vi "Process Heartbeat Waveform.vi"(7 "Pressure Measurement":dbl, 8 "error in (no error)":errorcluster, 11 "Heart Rate Params":T1={"Heart Rates"=[], "Peak Pressures"=[], "Peak Amplitudes"=[], "History Length"=20, "Last  Slope"=20.0, "filtered history"=[], "raw history"=[], "Pulse"=FALSE, "Heart Rate Timer"=0, "Iteration"=0, "Pressure of Valley"=0.0, "Slope Log"=[], "Signal Segment"=refnum, "Acquisition Graph"=refnum, "This VI"=refnum, "Name"=""}) -> (0 "error out":errorcluster, 1 "BPM":dbl, 2 "Last Slope":dbl(graph), 3 "Heart Rate Params Out":T1 caption="Heart Rate Params 2", 5 "Pulse":bool)   [LabVIEW 2017]
doc: "[Covers: SoftwareReq5]"
uses:
  Custom Controls/Heart Rate Parameters.ctl
panel:
  out "history":dbl[](array[numeric])
  out "Peak pressure":dbl
  out "Pressure":dbl
  out "Pressure low":dbl
  out "Slope":dbl
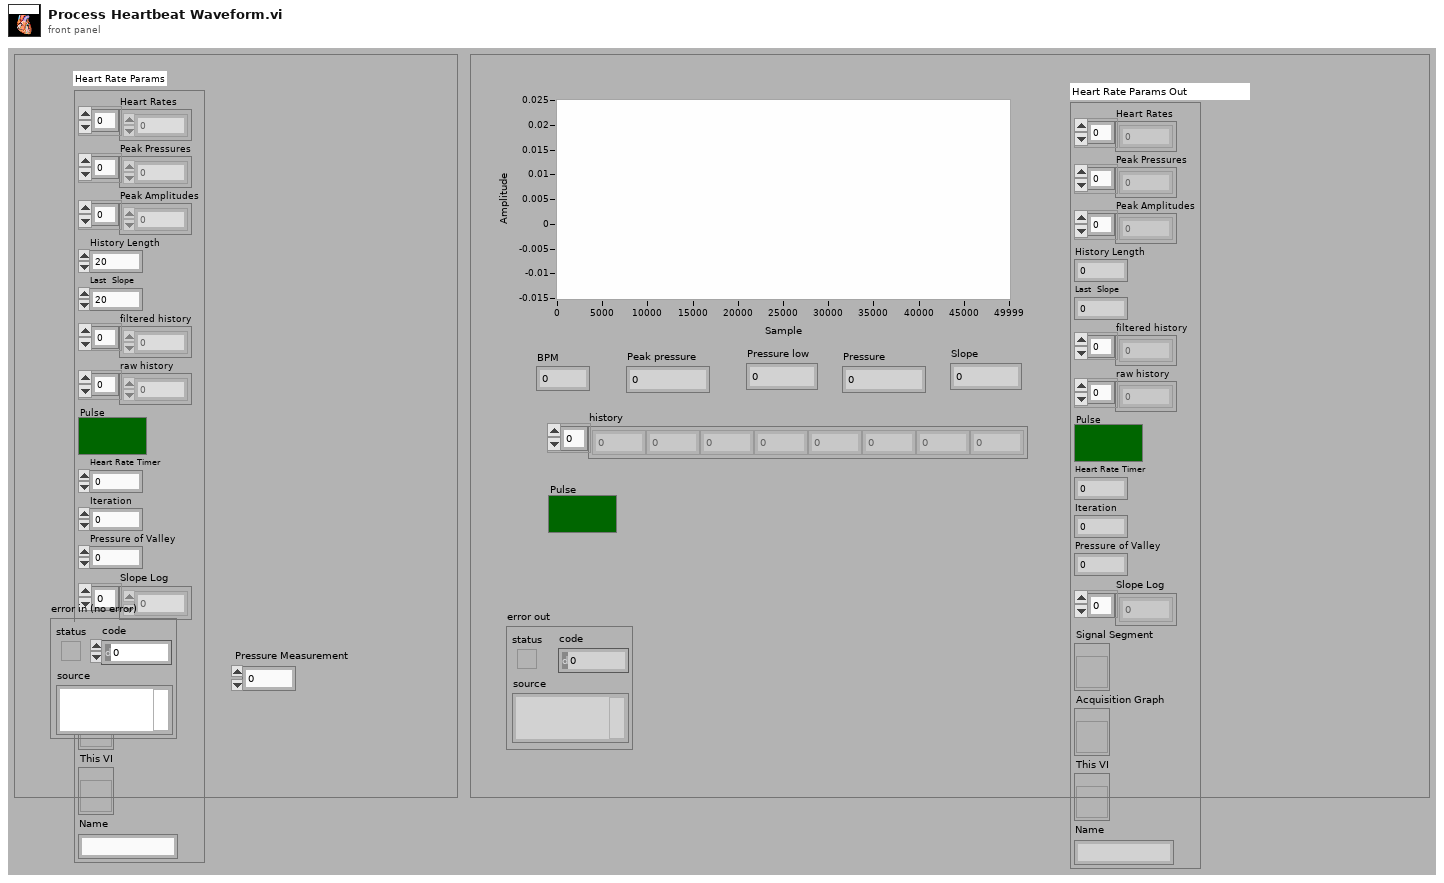
[diagram p1: front panel]
types:
  T1 = typedef "Heart Rate Parameters.ctl" = cluster{"Heart Rates":dbl[], "Peak Pressures":dbl[], "Peak Amplitudes":dbl[], "History Length":i32, "Last  Slope":dbl, "filtered history":dbl[], "raw history":dbl[], "Pulse":bool, "Heart Rate Timer":i32, "Iteration":u32, "Pressure of Valley":dbl, "Slope Log":dbl[], "Signal Segment":refnum<vi>, "Acquisition Graph":refnum<vi>, "This VI":refnum<vi>, "Name":string}
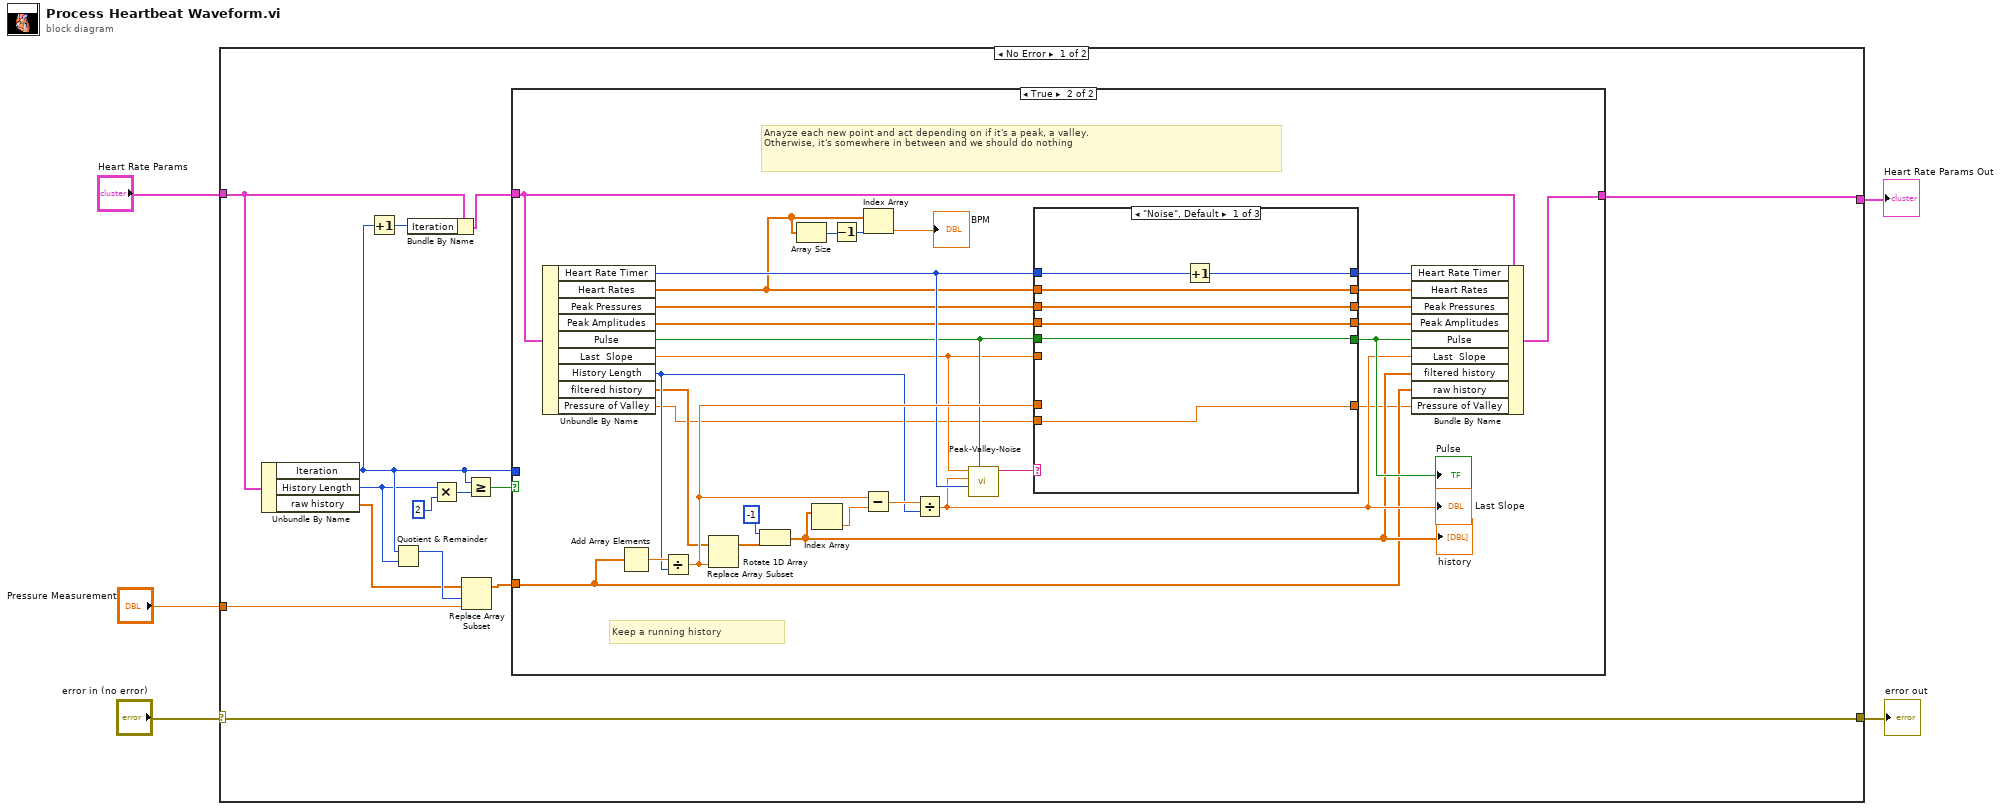
[diagram p0: block diagram]
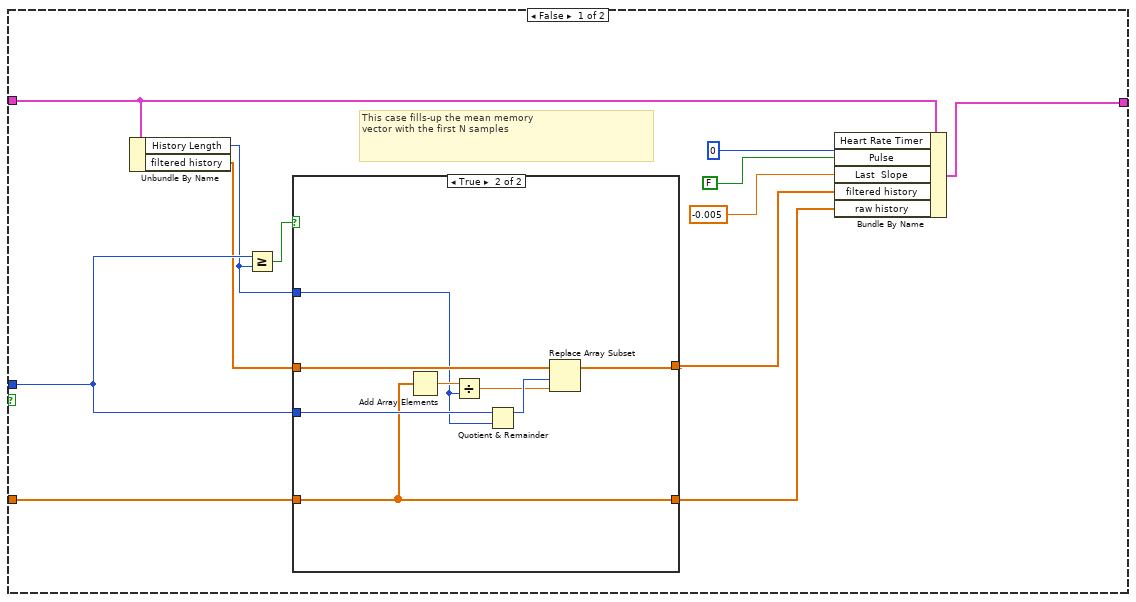
[diagram p2: hidden frame]
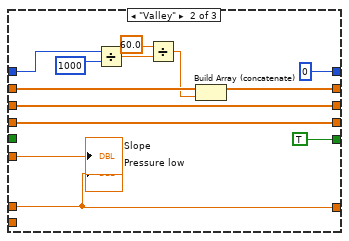
[diagram p4: hidden frame]
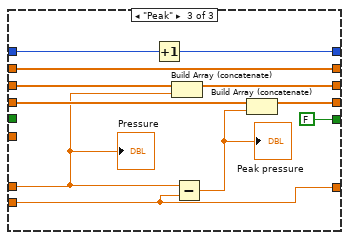
[diagram p5: hidden frame]
diagram:
  n1 = case shown="No Error" "error in (no error)" {
    selector: "error in (no error)" -> [w9 w104]
    tunnel: [w9 w104] -> w5
    tunnel: "Heart Rate Params" -> [w8 w103]
    tunnel: [w7 w103] -> w2
    tunnel: "Pressure Measurement" -> [w6 _]
    frame No Error {
      n2 = Unbundle By Name(w8) -> ("Iteration"=w16:u32, "History Length"=w10:i32, "raw history"=w13:dbl[])
      n3 = Increment(x=w16) -> (x+1=w14:u32)
      n4 = Quotient & Remainder(x=w16, y=w10) -> (x-y*floor(x/y)=w18:u32)  [unwired: 1 out]
      n5 = Bundle By Name(cluster=w8, "Iteration"=w14) -> (w15:T1)
      n6 = Multiply(x=w10, y=2) -> (x*y=w11:i32)
      n7 = Replace Array Subset(array=w13, new element=w6, index=w18) -> (w17:dbl[])
      n8 = Greater Or Equal?(x=w16, y=w11) -> (x >= y?=w19:bool)
      n9 = case shown="True" w19 {
        tunnel: w17 -> [w30 w50]
        tunnel: w16 -> [w29 _]
        tunnel: w15 -> [w24 w61]
        tunnel: [w28 w42] -> w7
        frame False {
          # "This case fills-up the mean memory \nvector with the first N samples"
          n10 = Unbundle By Name(w24) -> ("History Length"=w23:i32, "filtered history"=w21:dbl[])
          n11 = Greater Or Equal?(x=w29, y=w23) -> (x >= y?=w31:bool)
          n12 = case shown="True" w31 {
            tunnel: w30 -> [w33 w34]
            tunnel: w23 -> [_ w37]
            tunnel: w21 -> [w32 w39]
            tunnel: w29 -> [_ w38]
            tunnel: [w32 w35] -> w22
            tunnel: [w33 w34] -> w20
            frame False {
            }
            frame True {
              n13 = Add Array Elements(numeric array=w34) -> (sum=w41:dbl)
              n14 = Divide(x=w41, y=w37) -> (x/y=w36:dbl)
              n15 = Quotient & Remainder(x=w38, y=w37) -> (x-y*floor(x/y)=w40:u32)  [unwired: 1 out]
              n16 = Replace Array Subset(array=w39, new element=w36, index=w40) -> (w35:dbl[])
            }
          }
          n17 = Bundle By Name(cluster=w24, "Heart Rate Timer"=0, "Pulse"=FALSE, "Last  Slope"=-0.005, "filtered history"=w22, "raw history"=w20) -> (w28:T1)
        }
        frame True {
          # "Anayze each new point and act depending on if it's a peak, a valley.  \nOtherwise, it's somewhere in between and we should do nothing"
          # "Keep a running history"
          n18 = Unbundle By Name(w61) -> ("Heart Rate Timer"=w64:i32, "Heart Rates"=w46:dbl[], "Peak Pressures"=w63:dbl[], "Peak Amplitudes"=w62:dbl[], "Pulse"=w56:bool, "Last  Slope"=w55:dbl, "History Length"=w53:i32, "filtered history"=w51:dbl[], "Pressure of Valley"=w49:dbl)
          n19 = Add Array Elements(numeric array=w50) -> (sum=w71:dbl)
          n20 = Divide(x=w71, y=w53) -> (x/y=w65:dbl)
          n21 = Replace Array Subset(array=w51, new element=w65) -> (w69:dbl[])  [unwired: 1 in]
          n22 = Rotate 1D Array(1:w69, 2:-1 ("n")) -> (0:w52:dbl[])
          "history" <- w52
          n23 = Array Size(array=w46) -> (size(s)=w44:i32)
          n24 = Index Array(array=w52) -> (element=w68:dbl)  [unwired: 1 in]
          n25 = Decrement(x=w44) -> (x-1=w45:i32)
          n26 = Subtract(x=w65, y=w68) -> (x-y=w67:dbl)
          n27 = Index Array(array=w46, index=w45) -> (element=→"BPM":dbl)
          n28 = Divide(x=w67, y=w53) -> (x/y=w54:dbl)
          "Last Slope" <- w54
          n29 = call "Peak-Valley-Noise.vi"("Pulse"=w56, "Heart Rate Timer"=w64, "Slope"=w54, "Last Slope"=w55) -> ("State"=w66:string)  [unwired: 6 in, 1 out]
          n30 = case shown="\"Noise\", Default" w66 {
            tunnel: [w77 0 w102] -> w60
            tunnel: w64 -> [w78 w86 w100]
            tunnel: [w76 TRUE FALSE] -> w57
            tunnel: w56 -> [w76 _ _]
            tunnel: w55 -> [_ w87 _]
            tunnel: w65 -> [_ w79 w95]
            tunnel: w62 -> [w75 w89 w99]
            tunnel: w63 -> [w74 w88 w96]
            tunnel: [w74 w88 w94] -> w59
            tunnel: [w75 w89 w97] -> w58
            tunnel: w46 -> [w73 w82 w93]
            tunnel: [w73 w80 w93] -> w47
            tunnel: w49 -> [w72 _ w92]
            tunnel: [w72 w79 w92] -> w48
            frame "Noise", Default {
              n31 = Increment(x=w78) -> (x+1=w77:i32)
            }
            frame "Valley" {
              n32 = Divide(x=w86, y=1000) -> (x/y=w84:dbl)
              n33 = Divide(x=60.0, y=w84) -> (x/y=w81:dbl)
              n34 = Build Array (concatenate)(w82, w81) -> (w80:dbl[])
              "Slope" <- w87
              "Pressure low" <- w79
            }
            frame "Peak" {
              n35 = Increment(x=w100) -> (x+1=w102:i32)
              n36 = Build Array (concatenate)(w96, w95) -> (w94:dbl[])
              n37 = Subtract(x=w95, y=w92) -> (x-y=w98:dbl)
              "Peak pressure" <- w98
              n38 = Build Array (concatenate)(w99, w98) -> (w97:dbl[])
              "Pressure" <- w95
            }
          }
          "Pulse" <- w57
          n39 = Bundle By Name(cluster=w61, "Heart Rate Timer"=w60, "Heart Rates"=w47, "Peak Pressures"=w59, "Peak Amplitudes"=w58, "Pulse"=w57, "Last  Slope"=w54, "filtered history"=w52, "raw history"=w50, "Pressure of Valley"=w48) -> (w42:T1)
        }
      }
    }
    frame Error {
    }
  }
  "error out" <- w5
  "Heart Rate Params Out" <- w2
